vi "Draw BG Image.vi"(6 "Control Ref Queue":T4, 8 "error in (no error)":errorcluster, 10 "Multiplot Representation In":T1, 11 "2D Compass.lvclass in":refnum<class "2D Compass.lvclass">) -> (0 "error out":errorcluster, 2 "Multiplot Representation Out":T1, 3 "2D Compass.lvclass out":refnum<class "2D Compass.lvclass">)   [LabVIEW 2020, in "2D Compass.lvclass"]
uses:
  <vilib>/Math Plots/2D Math Plots/2D Compass/2D Compass/2D Compass.lvclass
  <vilib>/Math Plots/2D Math Plots/2D Plot/Action String/2DMathPlot Ctrl Act Queue.ctl
  <vilib>/Math Plots/2D Math Plots/2D Plot/Action String/2DMathPlot Ctrl Act Cluster.ctl
  <vilib>/Math Plots/2D Math Plots/2D Plot/Action String/2DMathPlot State Class.ctl
  e:/builds/penguin/labview/branches/2020/dev/dist/vi.lib/Math Plots/2D Math Plots/2D Plot/2D Plot/2D Plot.lvclass
  <vilib>/Math Plots/2D Math Plots/2D Plot/2D Plot/Typedef/Multiplot Representation.ctl
  <vilib>/Math Plots/2D Math Plots/2D Plot/2D Plot/Typedef/Plot Representation.ctl
  <vilib>/Math Plots/2D Math Plots/2D Plot/2D Plot/Typedef/Range Cluster.ctl
  <vilib>/Math Plots/2D Math Plots/2D Compass/2D Compass/2D Compass.lvclass/2D Compass.ctl
  <vilib>/Math Plots/2D Math Plots/2D Compass/2D Compass/Typedef/2D Compass Property.ctl
  <vilib>/Math Plots/2D Math Plots/2D Plot/2D Plot/2D Plot.lvclass
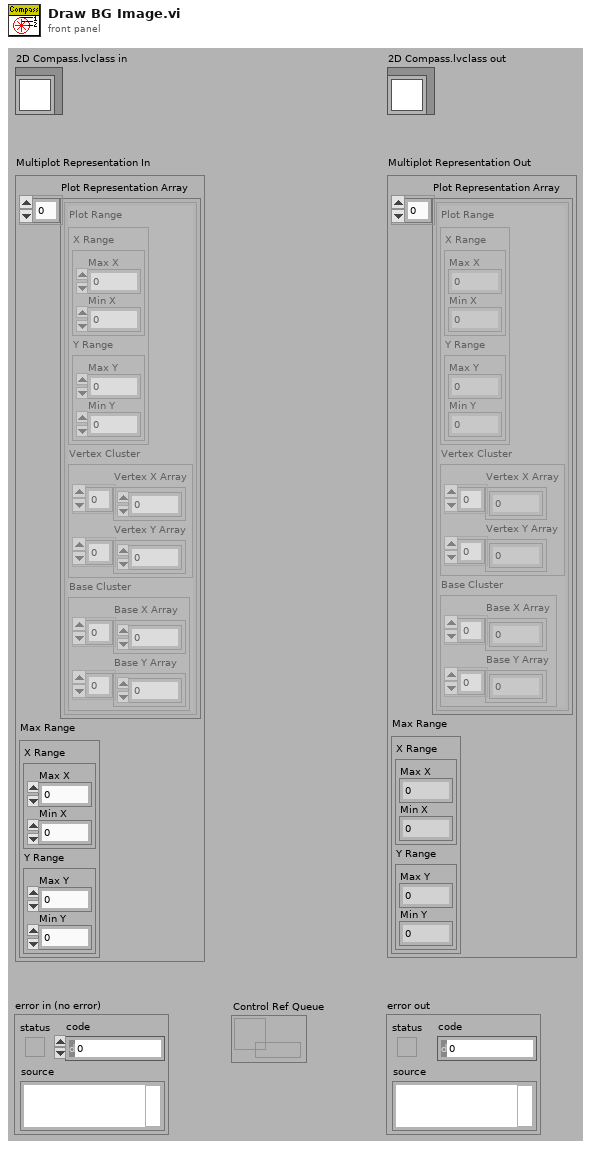
[diagram p1: front panel]
types:
  T1 = typedef "2D Plot.lvclass/Multiplot Representation.ctl" = cluster{"Plot Representation Array":T2[], "Max Range":T3}
  T2 = typedef "2D Plot.lvclass/Plot Representation.ctl" = cluster{"Plot Range":T3, "Vertex Cluster":cluster{"Vertex X Array":dbl[], "Vertex Y Array":dbl[]}, "Base Cluster":cluster{"Base X Array":dbl[], "Base Y Array":dbl[]}}
  T3 = typedef "2D Plot.lvclass/Range Cluster.ctl" = cluster{"X Range":cluster{"Max X":dbl, "Min X":dbl}, "Y Range":cluster{"Max Y":dbl, "Min Y":dbl}}
  T4 = typedef "2DMathPlot Ctrl Act Queue.ctl" = refnum<queue>
  T5 = typedef "2D Plot.lvclass/Property Cluster.ctl" = cluster{"Graph General":T6, "Format Property":string[], "Scale Array":T7, "Cursor Property":T10, "Annotation List":T12, "Active Cursor":i32, "Active Plot":i32}
  T6 = typedef "2D Plot.lvclass/Graph General Property.ctl" = cluster{"Palette Visible":cluster{"Graph Legend":bool, "Plot Legend":bool, "Auto size":bool, "Number of Plots":u32, "X Scrollbar":bool, "Scale Legend":bool, "Cursor Legend":bool}, "Plot Area Color":cluster{"FG Color":u32, "BG Color":u32}, "Bounds Size":cluster{"Width":u32, "Height":u32}, "Plot Area Bounds":cluster{"Left":i16, "Top":i16, "Right":i16, "Bottom":i16}}
  T7 = typedef "2D Plot.lvclass/Scale Array.ctl" = T8[]
  T8 = typedef "2D Plot.lvclass/Scale Cluster.ctl" = cluster{"General":cluster{"Editable":bool, "Flipped":bool, "Mapping Mode":u8, "Visible":bool, "Style":u8, "Scale Fit":u8}, "Offset and Multiplier":T9, "Range":cluster{"Minimum":dbl, "Maximum":dbl, "Increment":dbl, "Minor Increment":dbl, "Start":dbl}, "Tick Color":cluster{"Major Color":u32, "Minor Color":u32}, "Gird Color":cluster{"Major Color":u32, "Minor Color":u32}, "Marker":cluster{"Visible":bool, "FG Color":u32, "BG Color":u32, "Font Name":string, "Font Size":u32, "Font Bold":bool, "Font Italic":bool, "Font Strikeout":bool, "Font Underline":bool}, "Name Label":cluster{"Visible":bool, "FG Color":u32, "BG Color":u32, "Font Name":string, "Font Size":u32, "Font Bold":bool, "Font Italic":bool, "Font Strikeout":bool, "Font Underline":bool, "Justification":enum16{"Left", "Center", "Right"}, "Text":string}}
  T9 = typedef "LVOffsetAndMultiplierTypeDef.ctl" = cluster{"Offset":dbl, "Multiplier":dbl}
  T10 = typedef "2D Plot.lvclass/Cursor Property.ctl" = cluster{"Cursor List":T11, "Cursor List Addtional":cluster{"Cursor Selection Color":u32, "Line Style":u8, "Line Width":u8, "Visible":bool}[]}
  T11 = typedef "LVCursorListTypeDef.ctl" = cluster{"Name":string, "Color":u32, "Style":u8, "Point Style":u8, "Name Visible":bool, "Allow Drag":bool, "Cursor Mode":u32, "Plot":i32, "Index":i32, "Position":cluster{"X":dbl, "Y":dbl}, "X Scale":u32, "Y Scale":u32, "Watch Plots":i32[], "Watch All Plots":bool, "Plot Area":i32, "Label Offset":cluster{"X":dbl, "Y":dbl}}[]
  T12 = typedef "LVAnnotationListTypeDef.ctl" = cluster{"Name":string, "Color":u32, "Style":u8, "Point Style":u8, "Name Visible":bool, "Allow Drag":bool, "Annotation Mode":u32, "Plot":i32, "Index":i32, "Position":cluster{"X":dbl, "Y":dbl}, "X Scale":u32, "Y Scale":u32, "Show Arrow":bool, "Lock Name":bool, "Plot Area":i32, "Label Offset":cluster{"X":dbl, "Y":dbl}}[]
  T13 = typedef "2D Plot.lvclass/Plot Property Array.ctl" = T14[]
  T14 = typedef "2D Plot.lvclass/Plot Property.ctl" = cluster{"Bar Plot Style":u8, "DigitalLineStyle":u8, "TransitionLocation":u8, "Transition Type":u8, "Fill To":i16, "Fill/Pt. Color":u32, "Label Style":u8, "Line Style":u8, "Line Width":u8, "Plot Color":u32, "Plot Interpolation":u8, "Plot Name":string, "Point Style":u8, "Visible?":bool, "XScaleIdx":u32, "YScaleIdx":u32}
  T15 = typedef "2D Compass.lvclass/2D Compass Property Array.ctl" = T16[]
  T16 = typedef "2D Compass.lvclass/2D Compass Property.ctl" = cluster{"Compass Size":dbl}
  T17 = cluster{"Plot Property Array":T13, "2D Compass Array":T15, "Scale Visibility":cluster{"Phase Scale":bool}}
  T18 = typedef "2DMathPlot Ctrl Act Cluster.ctl" = cluster{"Plot Area Ref":refnum<vi>, "Z Axis Ref":refnum<vi>, "Legend Ref":refnum<vi>, "XControl Ref":refnum<vi>, "Facade Ref":refnum<vi>, "Display State Change Class":T19}
  T19 = typedef "2DMathPlot State Class.ctl" = enum16{"Update All (Undo)", "Update General", "Update Appearance", "Update Format", "Update Scale", "Update Marker", "Update Cursor", "None"}
  T20 = cluster{"Left":i32, "Top":i32, "Right":i32, "Bottom":i32}
  T21 = typedef "LVPoint32TypeDef.ctl" = cluster{"Horizontal":i32, "Vertical":i32}
  T22 = cluster{"left":i32, "top":i32, "right":i32, "bottom":i32}
  T23 = typedef "2D Compass.lvclass/BG Image Property.ctl" = cluster{"Radius":i16[], "Plot Area Bounds":T24, "Center position":cluster{"X":i16, "Y":i16}, "Flip?":bool, "Major Gird Color":u32, "Minor Gird Color":u32}
  T24 = typedef "LVRectTypeDef.ctl" = cluster{"Left":i16, "Top":i16, "Right":i16, "Bottom":i16}
  T25 = cluster{"Width":u16, "Style":enum32{"Solid", "Dash", "Dot", "DashDot", "DashDotDot"}}
  T26 = cluster{"Vertex X Array":dbl[], "Vertex Y Array":dbl[]}
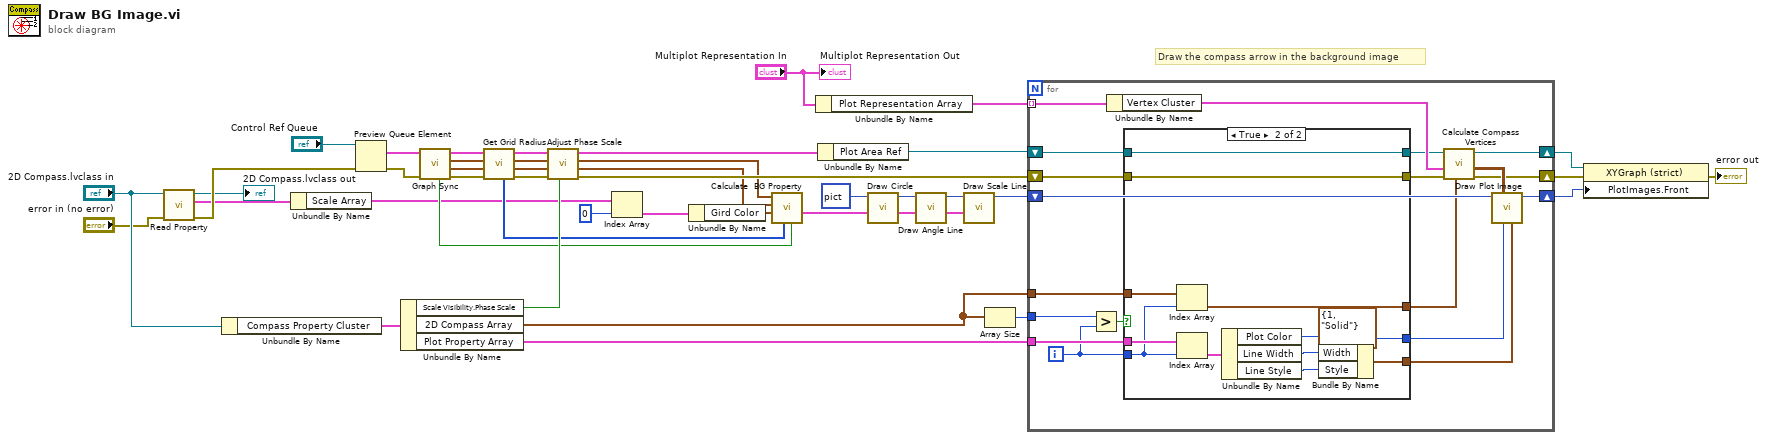
[diagram p0: block diagram]
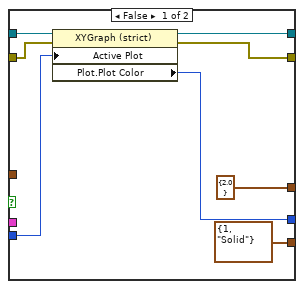
[diagram p2: hidden frame]
diagram:
  # "Draw the compass arrow in the background image"
  n1 = call <vilib>:"Read Property.vi"("error in (no error)"="error in (no error)", "2D Plot.lvclass in"="2D Compass.lvclass in") -> ("error out"=w9:errorcluster, "XY Graph Property Cluster"=w5:T5, "2D Plot.lvclass out"=→"2D Compass.lvclass out":refnum<class "2D Compass.lvclass">)  [unwired: 7 out]
  n2 = Unbundle By Name("2D Compass.lvclass in") -> ("Compass Property Cluster"=w25:T17)
  n3 = Unbundle By Name(w5) -> ("Scale Array"=w8:T7)
  n4 = Preview Queue Element(queue="Control Ref Queue", error in (no error)=w9) -> (element=w19:T18, error out=w26:errorcluster)  [unwired: 3 out]
  n5 = Unbundle By Name(w25) -> ("Scale Visibility.Phase Scale"=w34:bool, "2D Compass Array"=w28:T15, "Plot Property Array"=w31:T13)
  n6 = call <vilib>:"Graph Sync.vi"("error in (no error)"=w26, "Control Ref Cluster"=w19) -> ("error out"=w20:errorcluster, "Plot Area Bounds"=w17:T20, "Origin Coords"=w21:T21, "Dup Control Ref Cluster"=w44:T18, "Flip?"=w14:bool)  [unwired: 1 in, 4 out]
  n7 = call <vilib>:"Get Grid Radius.vi"("error in (no error)"=w20, "Origin Coords"=w21, "Control Ref Cluster"=w44) -> ("error out"=w36:errorcluster, "Dup Origin Coords"=w18:T21, "Dup Control Ref Cluster"=w16:T18, "Radius Array"=w22:i16[])  [unwired: 1 in, 4 out]
  n8 = call <vilib>:"Adjust Phase Scale.vi"("Show Scale?"=w34, "error in (no error)"=w36, "Plot Area Bounds"=w17, "Origin Coords"=w18, "Control Ref Cluster"=w16) -> ("error out"=w13:errorcluster, "Dup Plot Area Bounds"=w3:T22, "Dup Origin Coords"=w4:T21, "Dup Control Ref Cluster"=w12:T18)  [unwired: 3 out]
  n9 = Index Array(array=w8, index=0) -> (element=w7:T8)
  n10 = Unbundle By Name(w7) -> ("Gird Color"=w6:cluster{"Major Color":u32, "Minor Color":u32})
  n11 = call <vilib>:"Calculate  BG Property.vi"("Flip?"=w14, "Radius Array"=w22, "Gird Color"=w6, "Plot Area Bounds"=w3, "Zero Point Coords"=w4) -> ("BG Image Property"=w43:T23)  [unwired: 3 in, 3 out]
  n12 = Unbundle By Name("Multiplot Representation In") -> ("Plot Representation Array"=w23:T2[])
  n13 = Unbundle By Name(w12) -> ("Plot Area Ref"=w15:refnum<vi>)
  n14 = call <vilib>:"Draw Circle.vi"("BG Image Property In"=w43, "Picture In"=picture data[5B]) -> ("BG Image Property Out"=w38:T23, "Picture Out"=w41:picture)  [unwired: 8 out]
  n15 = call <vilib>:"Draw Angle Line.vi"("BG Image Property In"=w38, "Picture In"=w41) -> ("BG Image Property Out"=w39:T23, "Picture Out"=w40:picture)  [unwired: 8 out]
  n16 = call <vilib>:"Draw Scale Line.vi"("BG Image Property In"=w39, "Picture In"=w40) -> ("Picture Out"=w33:picture)  [unwired: 9 out]
  n17 = Array Size(array=w28) -> (size(s)=w27:i32)
  n18 = for {
    shift-right: [w60] -> w32
    shift-left: w33 -> [w61]
    tunnel: w31 -> [w63]
    tunnel: w28 -> [w62]
    shift-right: [w57] -> w30
    shift-left: w15 -> [w48]
    shift-right: [w56] -> w29
    shift-left: w13 -> [w46]
    tunnel: w27 -> [w53]
    tunnel: w23 -> [w50] mode=indexing
    i -> [w52]
    n19 = Greater?(x=w53, y=w52) -> (0:w51:bool)
    n20 = Unbundle By Name(w50) -> ("Vertex Cluster"=w49:T26)
    n21 = case shown="True" w51 {
      tunnel: w63 -> [_ w83]
      tunnel: w62 -> [_ w82]
      tunnel: [T16 {"Compass Size"=2.0} w81] -> w59
      tunnel: [w67 w77] -> w55
      tunnel: [T25 {"Width"=1, "Style"=enum."Solid"} ("pen") w76] -> w54
      tunnel: w52 -> [w66 w74]
      tunnel: w48 -> [w69 w73]
      tunnel: [w68 w73] -> w47
      tunnel: w46 -> [w65 w72]
      tunnel: [w64 w72] -> w45
      frame False {
        n22 = property class="XYGraph (strict)"(reference=w69, error in=w65, "Active Plot"=w66) -> (reference out=w68:refnum<vi>, error out=w64:errorcluster, "Plot.Plot Color"=w67:u32)
      }
      frame True {
        n23 = Index Array(array=w82, index=w74) -> (element=w81:T16)
        n24 = Index Array(array=w83, index=w74) -> (element=w78:T14)
        n25 = Unbundle By Name(w78) -> ("Plot Color"=w77:u32, "Line Width"=w80:u8, "Line Style"=w79:u8)
        n26 = Bundle By Name(cluster=T25 {"Width"=1, "Style"=enum."Solid"} ("pen"), "Width"=w80, "Style"=w79) -> (w76:T25)
      }
    }
    n27 = call <vilib>:"Calculate Compass Vertices.vi"("2D Compass Property"=w59, "error in (no error)"=w45, "Vertex Cluster"=w49, "Polar Area Ref In"=w47) -> ("error out"=w56:errorcluster, "Compass Vertex"=w58:cluster{"X":i16, "Y":i16}[][], "Polar Area Ref Out"=w57:refnum<vi>)  [unwired: 1 in, 4 out]
    n28 = call <vilib>:"Draw Plot Image.vi"("pen"=w54, "Plot Color"=w55, "Plot Vertex"=w58, "Picture In"=w61) -> ("Picture Out"=w60:picture)  [unwired: 1 in, 6 out]
  }
  n29 = property class="XYGraph (strict)"(reference=w30, error in=w29, "PlotImages.Front"=w32) -> (error out=→"error out":errorcluster)  [unwired: 1 out]
  "Multiplot Representation Out" <- "Multiplot Representation In"
